vi "Dialog Display.vi"() -> ()   [LabVIEW 2018]
panel:
  in  "stop":bool
  in  "Boolean":bool
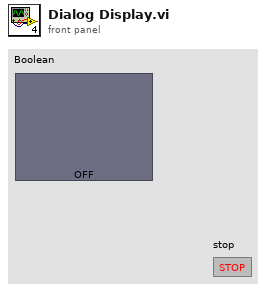
[diagram p1: front panel]
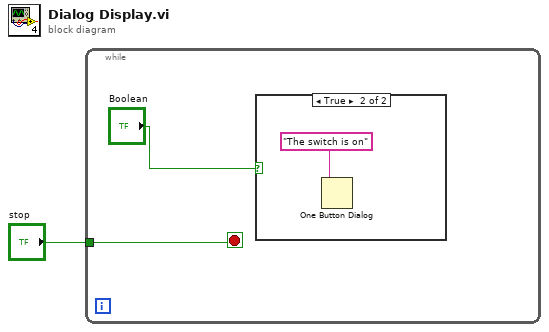
[diagram p0: block diagram]
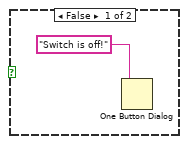
[diagram p2: hidden frame]
diagram:
  n1 = while {
    tunnel: "stop" -> [w2]
    stop <- w2 stop-if-true
    n2 = case shown="True" "Boolean" {
      frame False {
        n3 = One Button Dialog(message="Switch is off!") -> ()  [unwired: 1 in, 1 out]
      }
      frame True {
        n4 = One Button Dialog(message="The switch is on") -> ()  [unwired: 1 in, 1 out]
      }
    }
  }
